vi "SubTemplate_GetAttributesToModify.vi"(0 "reference in":refnum<class "SubTemplate.lvclass">, 3 "timeout (15000 ms)":i32=15000, 5 "error in (no error)":errorcluster) -> (14 "reference out":refnum<class "SubTemplate.lvclass">, 16 "Attributes":T1 {"Base class"."Attribute1" format="%.2f"}, 17 "Timeout":bool, 19 "error out":errorcluster)   [LabVIEW 2012, in "SubTemplate.lvclass"]
doc: "This VI returns the attributes associated with this object reference and places a lock on the object.\n\nIf the object is currently locked for modification by another method, 'Timeout' specifies how long the VI should wait to receive access to the object. The default value waits until the object becomes available.\n\nYou must use this class SetModifiedAttributes VI to set the object's data and release the lock."
uses:
  <resource>/Framework/Providers/Open_GDS/ClassProviders/Provider_EndevoGOOP300/Templates/SubTemplate/SubTemplate.lvclass
  <resource>/Framework/Providers/Open_GDS/ClassProviders/Provider_EndevoGOOP300/Templates/SubTemplate/protected/ObjectAttributes.ctl
  <resource>/Framework/Providers/Open_GDS/ClassProviders/Provider_EndevoGOOP300/Templates/BaseTemplate/protected/ObjectAttributes.ctl
  <vilib>/addons/_goop3.llb/3GOOPStates.ctl
  <resource>/Framework/Providers/Open_GDS/ClassProviders/Provider_EndevoGOOP300/Templates/SubTemplate/SubTemplate.lvclass/SubTemplate.ctl
  <resource>/Framework/Providers/Open_GDS/ClassProviders/Provider_EndevoGOOP300/Templates/BaseTemplate/BaseTemplate.lvclass
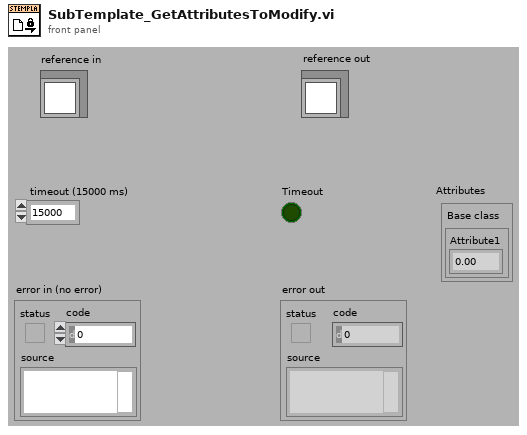
[diagram p1: front panel]
types:
  T1 = typedef "SubTemplate.lvclass/ObjectAttributes.ctl" = cluster{"Base class":T2}
  T2 = typedef "BaseTemplate.lvclass/ObjectAttributes.ctl" = cluster{"Attribute1":dbl}
  T3 = typedef "3GOOPStates.ctl" = enum16{"Set", "Get", "New", "Delete", "Clear", "Test and get", "Unlock data", "Information", "Look up existing", "New or look up existing", "Test and get shared", "Get shared", "Set shared", "Unlock shared", "Find dynamic method", "Register dynamic method", "Preload dynamic method", "Probe", "Cast to more generic", "Cast to more specific"}
  T4 = typedef "BaseTemplate.lvclass/ObjectReference.ctl" = refnum<k1>
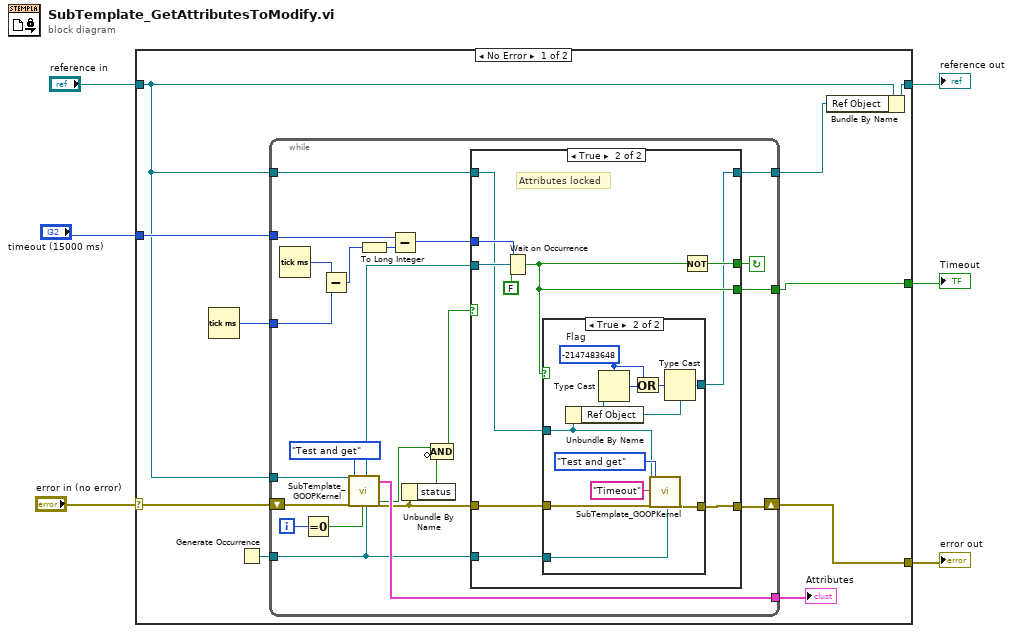
[diagram p0: block diagram]
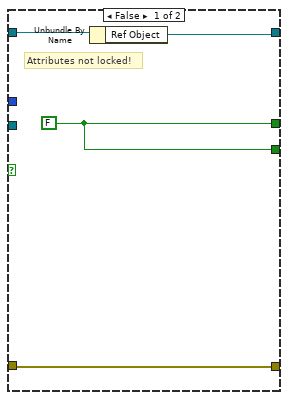
[diagram p2: hidden frame]
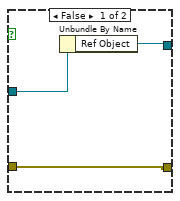
[diagram p3: hidden frame]
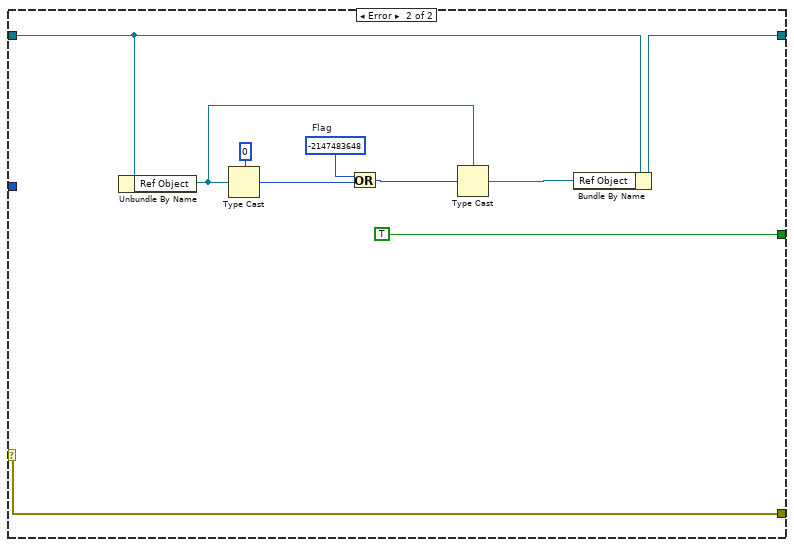
[diagram p4: hidden frame]
diagram:
  n1 = case shown="No Error" "error in (no error)" {
    selector: "error in (no error)" -> [w13 w77]
    tunnel: [w10 w73] -> w3
    tunnel: [w12 w77] -> w1
    tunnel: "reference in" -> [w8 w74]
    tunnel: [w11 TRUE ("timed out")] -> w2
    tunnel: "timeout (15000 ms)" -> [w14 _]
    frame No Error {
      n2 = Tick Count (ms)() -> (millisecond timer value=w15:u32)
      n3 = Generate Occurrence() -> (w16:refnum<k4>)
      n4 = while {
        tunnel: [w35] -> w9
        shift-left: w13 -> [w36]
        shift-right: [w21] -> w12
        tunnel: [w38] -> w11
        tunnel: w14 -> [w27]
        tunnel: w8 -> [w37]
        tunnel: w16 -> [w20]
        tunnel: w15 -> [w17]
        tunnel: w8 -> [w23]
        tunnel: [w19] -> w7
        i -> [w31]
        stop <- w39 continue-if-true
        n5 = Tick Count (ms)() -> (millisecond timer value=w18:u32)
        n6 = Equal To 0?(x=w31) -> (x = 0?=w30:bool)
        n7 = Subtract(x=w18, y=w17) -> (x-y=w26:u32)
        n8 = call <resource>:"SubTemplate_GOOPKernel.vi"("Ref in"=w37, "error in (no error)"=w36, "Action"=3GOOPStates."Test and get", "Misc"=w30, "Occurrence"=w20) -> ("Occurrence out"=w29:refnum<k4>, "Data out"=w35:T1, "Data locked?"=w33:bool, "error out"=w22:errorcluster)  [unwired: 12 in, 7 out]
        n9 = To Long Integer(number=w26) -> (32bit integer=w24:i32)
        n10 = Subtract(x=w27, y=w24) -> (x-y=w25:i32)
        n11 = Unbundle By Name(w22) -> ("status"=w34:bool)
        n12 = Compound Arithmetic op=AND(w33, invert w34) -> (w32:bool)
        n13 = case shown="True" w32 {
          tunnel: w29 -> [_ w52]
          tunnel: w25 -> [_ w50]
          tunnel: [w43 w53] -> w39
          tunnel: [w43 w46] -> w38
          tunnel: w23 -> [w41 w49]
          tunnel: w22 -> [w42 w48]
          tunnel: [w42 w47] -> w21
          tunnel: w20 -> [_ w45]
          tunnel: [w40 w44] -> w19
          frame False {
            w43 = FALSE
            # "Attributes not locked!"
            n14 = Unbundle By Name(w41) -> ("Ref Object"=w40:T4)
          }
          frame True {
            # "Attributes locked"
            n15 = Wait on Occurrence(1:FALSE ("ignore previous (T)"), 2:w52, 3:w50) -> (0:w46:bool)
            n16 = case shown="True" w46 {
              tunnel: w49 -> [w55 w62]
              tunnel: w48 -> [w56 w67]
              tunnel: [w56 w66] -> w47
              tunnel: w45 -> [_ w64]
              tunnel: [w54 w57] -> w44
              frame False {
                n17 = Unbundle By Name(w55) -> ("Ref Object"=w54:T4)
              }
              frame True {
                w61 = -2147483648  # Flag
                n18 = Unbundle By Name(w62) -> ("Ref Object"=w58:T4)
                n19 = Type Cast(type=w61, x=w58) -> (*(type *) &x=w60:i32)
                n20 = Or(x=w61, y=w60) -> (x .or. y?=w59:i32)
                n21 = call <resource>:"SubTemplate_GOOPKernel.vi"("Ref in"=w62, "Probe in"="Timeout" ("VI ref"), "error in (no error)"=w67, "Action"=3GOOPStates."Test and get", "Occurrence"=w64) -> ("error out"=w66:errorcluster)  [unwired: 12 in, 10 out]
                n22 = Type Cast(type=w58, x=w59) -> (*(type *) &x=w57:T4)
              }
            }
            n23 = Not(x=w46) -> (.not. x?=w53:bool)
          }
        }
      }
      "Attributes" <- w9
      n24 = Bundle By Name(cluster=w8, "Ref Object"=w7) -> (w10:refnum<class "SubTemplate.lvclass">)
    }
    frame Error {
      w75 = -2147483648  # Flag
      n25 = Unbundle By Name(w74) -> ("Ref Object"=w68:T4)
      n26 = Type Cast(type=0, x=w68) -> (*(type *) &x=w71:i32)
      n27 = Or(x=w75, y=w71) -> (x .or. y?=w70:i32)
      n28 = Type Cast(type=w68, x=w70) -> (*(type *) &x=w69:T4)
      n29 = Bundle By Name(cluster=w74, "Ref Object"=w69) -> (w73:refnum<class "SubTemplate.lvclass">)
    }
  }
  "error out" <- w1
  "reference out" <- w3
  "Timeout" <- w2
